vi "truncate to 48bits.vi"() -> ()   [LabVIEW 2020]
panel:
  out "x*y":i32
  out "Array":u8[](array[numeric]) format="%x"
  out "text":string
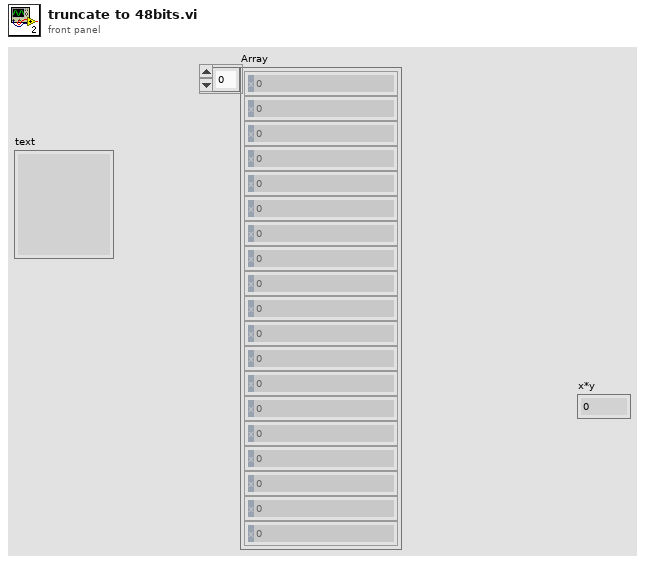
[diagram p1: front panel]
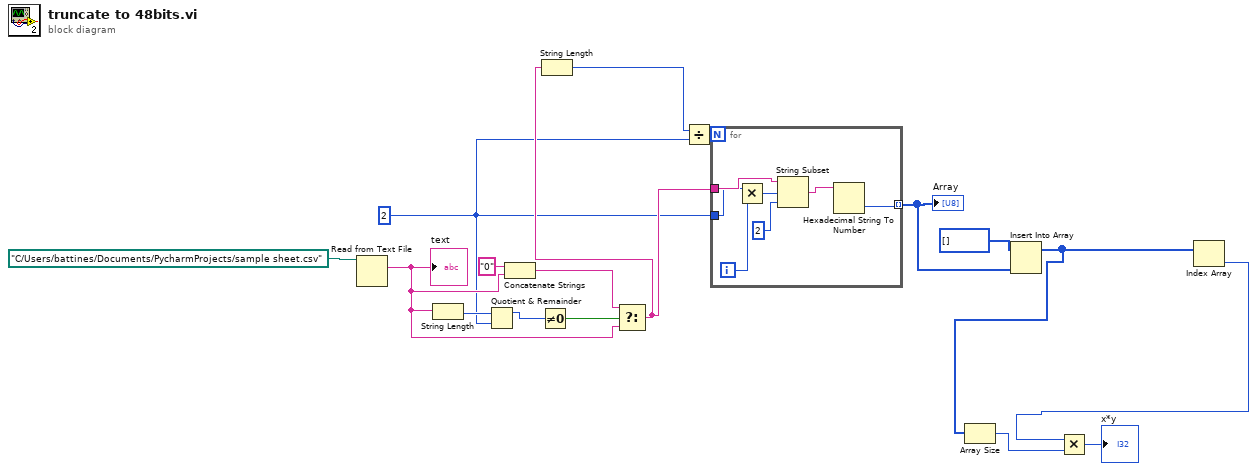
[diagram p0: block diagram]
diagram:
  w7 = 2 ("x")
  n1 = Read from Text File(file (use dialog)=path "C:/Users/battines/Documents/PycharmProjects/sample sheet.csv") -> (text=w11:string)  [unwired: 3 in, 3 out]
  "text" <- w11
  n2 = String Length(string=w11) -> (length=w15:i32)
  n3 = Quotient & Remainder(x=w15, y=w7) -> (x-y*floor(x/y)=w14:i32)  [unwired: 1 out]
  n4 = Concatenate Strings("0" ("string"), w11) -> (w12:string)
  n5 = Not Equal To 0?(x=w14) -> (x != 0?=w13:bool)
  n6 = Select(t=w12, s=w13, f=w11) -> (s? t:f=w8:string)
  n7 = String Length(string=w8) -> (length=w9:i32)
  n8 = Divide(x=w9, y=w7) -> (x/y=w10:dbl)
  n9 = for {
    N: w10 -> [_]
    tunnel: w8 -> [w20]
    tunnel: [w21] -> w6 mode=indexing
    tunnel: w7 -> [w19]
    i -> [w23]
    n10 = Multiply(x=w19, y=w23) -> (x*y=w24:i32)
    n11 = String Subset(string=w20, offset (0)=w24, length (rest)=2 ("length (rest)")) -> (substring=w22:string)
    n12 = Hexadecimal String To Number(string=w22) -> (number=w21:u32)  [unwired: 2 in, 1 out]
  }
  "Array" <- w6
  n13 = Insert Into Array(array=u8[] [], new element=w6) -> (w4:u8[])  [unwired: 1 in]
  n14 = Array Size(array=w4) -> (size(s)=w2:i32)
  n15 = Index Array(array=w4) -> (element=w3:u8)  [unwired: 1 in]
  n16 = Multiply(x=w3, y=w2) -> (x*y=→"x*y":i32)
